vi "Subscribe.vi"(8 "error in (no error)":errorcluster, 10 "Subscription Request":refnum<class "SubscriptionRequest.lvclass">, 11 "IMediator In":refnum<class "IMediator.lvclass">) -> (0 "error out":errorcluster, 3 "IMediator Out":refnum<class "IMediator.lvclass">)   [LabVIEW 2019, in "IMediator.lvlib" / "IMediator.lvclass"]
doc: "<License>\nCopyright © 2017 Composed Systems, LLC | All rights reserved\nwww.composed.io\n\nAuthor: Ethan Stern <ethan.stern@composed.io>\n\nThis software is provided \"AS IS\" WITHOUT WARRANTIES, either express or implied, AND IS FOR EDUCATIONAL PURPOSES ONLY.\n</License>"
uses:
  <vilib>/gpm_packages/@cs/mva-core/Source/IMediator/IMediator/IMediator.lvclass
  <vilib>/gpm_packages/@cs/mva-core/Source/IMediator/SubscriptionRequest/SubscriptionRequest.lvclass
panel:
  # "Who wants it? (Unique Subscriber ID)\nWhat do they want? (Datum Name and Type)\nWhere/how do they want it sent? (Transport)\nWhen/under what conditions? (SubscriptionPolicy)"
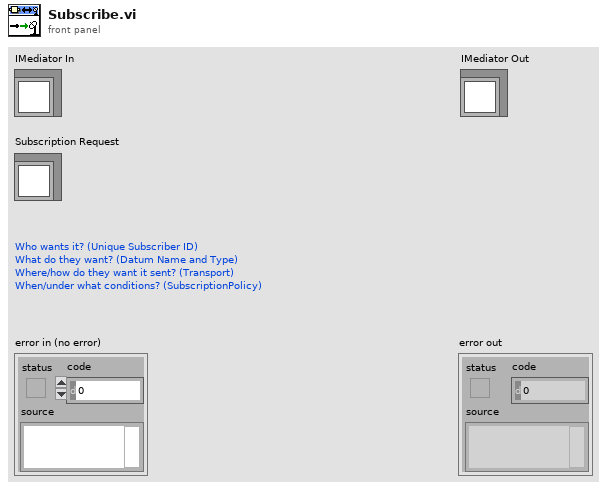
[diagram p1: front panel]
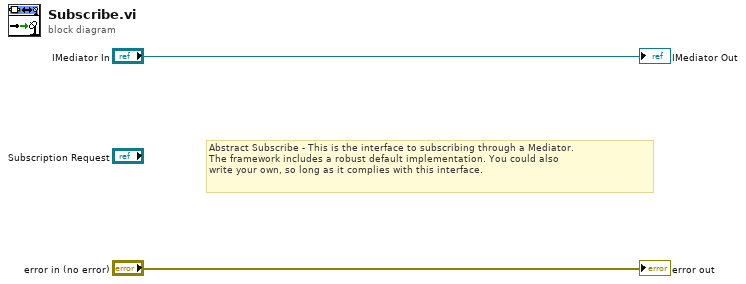
[diagram p0: block diagram]
diagram:
  # "Abstract Subscribe - This is the interface to subscribing through a Mediator.\nThe framework includes a robust default implementation. You could also\nwrite your own, so long as it complies with this interface."
  "error out" <- "error in (no error)"
  "IMediator Out" <- "IMediator In"
